vi "test.vi"() -> ()   [LabVIEW 2016]
panel:
  out "asdf":string
  in  "Stopp":bool
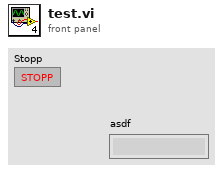
[diagram p1: front panel]
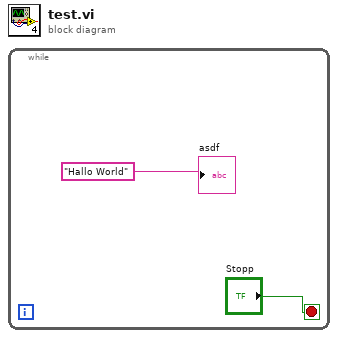
[diagram p0: block diagram]
diagram:
  n1 = while {
    stop <- "Stopp" stop-if-true
    "asdf" <- "Hallo World"
  }
